vi "u8.vi"(9 "idx":u8, 10 "data in":u8, 11 "Message Counter (U8)":u8) -> (3 "data out":u8)   [LabVIEW 2020]
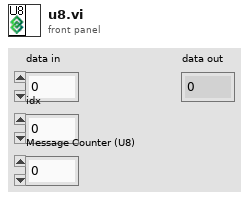
[diagram p1: front panel]
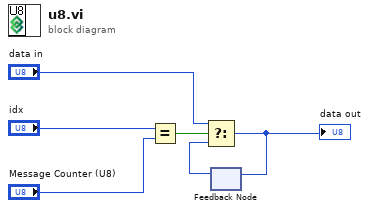
[diagram p0: block diagram]
diagram:
  n1 = Equal?(x="idx", y="Message Counter (U8)") -> (x = y?=w3:bool)
  n2 = feedback #1() -> (w5:u8)  [unwired: 1 in]
  n3 = Select(t="data in", s=w3, f=w5) -> (s? t:f=w6:u8)
  "data out" <- w6
  n4 = feedback-in #1(w6) -> ()
